vi "Generate Overlap SQL Query.vi"(8 "error in (no error)":errorcluster, 11 "Importing Transactions":refnum<class "Credit Statement.lvclass">) -> (0 "error out":errorcluster, 2 "Overlap Query":string, 3 "Overlapping Records":refnum<class "Statement.lvclass">)   [LabVIEW 2018, in "Credit Statement.lvclass"]
uses:
  Credit Statement.lvclass
  C:/Users/jtipps/Documents/Filthy-Lucre-Budgetizer/source/support/classes/Statement/Statement.lvclass
  Statement/Statement.lvclass
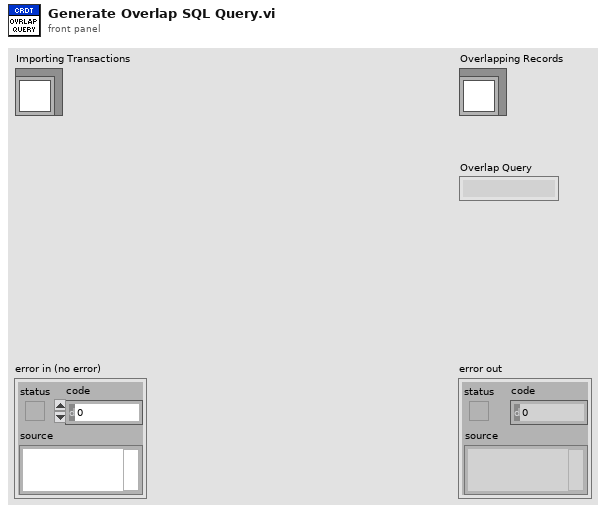
[diagram p1: front panel]
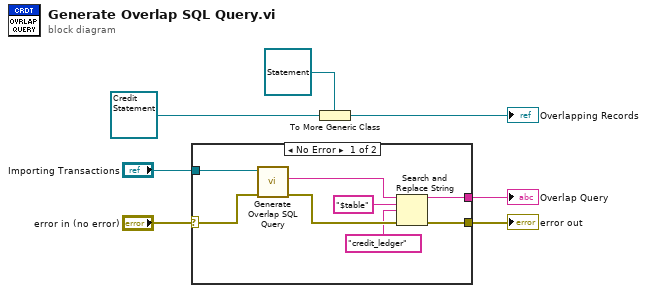
[diagram p0: block diagram]
diagram:
  n1 = case shown="No Error" "error in (no error)" {
    selector: "error in (no error)" -> [w8 w16]
    tunnel: "Importing Transactions" -> [w15 _]
    tunnel: [w10 w16] -> w5
    tunnel: [w9 _] -> w4
    frame No Error {
      n2 = call-parent "Generate Overlap SQL Query.vi"("error in (no error)"=w8, "Importing Transactions"=w15) -> ("error out"=w13:errorcluster, "Overlap Query"=w14:string)  [unwired: 7 in, 1 out]
      n3 = Search and Replace String(input string=w14, search string="$table", replace string="credit_ledger", error in=w13) -> (result string=w9:string, error out=w10:errorcluster)  [unwired: 4 in, 2 out]
    }
    frame Error {
    }
  }
  "error out" <- w5
  "Overlap Query" <- w4
  n4 = To More Generic Class(target class=refnum<class "Statement.lvclass"> refnum ("Overlapping Records"), reference=refnum<class "Credit Statement.lvclass"> refnum ("Credit Statement in")) -> (generic class reference=→"Overlapping Records":refnum<class "Statement.lvclass">)
